vi "LEMP_realtime_theory_object_update.vi"() -> ()   [LabVIEW 2021]
uses:
  <vilib>/gmath/NI_Gmath.lvlib
  <vilib>/gmath/statdist.llb/Normal Moments.vi
panel:
  in  "Eigenvalue Method":u16(ring) items=["0-Local Eigen Modification Procedure", "1-LabVIEW generalized eigenvalues", "2-LabVIEW M^-1K eigenvalues", "3-LabVIEW Cholesky Factorization", "4-Cholesky Factorization CPU SGL", "5-Cholesky Factorization CPU FXP", "6-Cholesky Factorization FPGA SGL", "7-Cholesky Factorization FPGA SGL SCL"]
  in  "Width":dbl=0.0508 min=0.0 format="%#.6f"
  in  "Density":dbl=7900.0
  in  "Height":dbl=0.00635
  in  "Length of Beam":dbl=0.3525
  in  "Young's Modulus":dbl=209500000000.0
  in  "Torsion Spring":dbl format="%#.6f"
  in  "Initial Pin node":i32
  in  "Std. Dev.":dbl=0.5 min=0.0
  in  "FFT data length (data points)":i32=5000
  in  "Min. FFT Power Value (RMS)":dbl=0.02
  in  "accelerometer_mass":dbl=0.055
  in  "Std. Dev = Number of Particles / 3":bool
  in  "Number Of Particles":i32=5 min=3 step=1
  in  "FEA Nodes":i32=40 min=10 max=500 step=1
  in  "File name":i32
  in  "Auto FFT length":bool
  in  "scaling_factor_Hz_per_pin_to_frequency_resolution":dbl=0.33 caption="Scale FFT Factor" format="%#_13g"
  in  "Save Acceleration Data":bool
  in  "Max Roller Velocity":dbl=3.32
  in  "Bound to 1st Frequency":bool=TRUE
  in  "Mode Count":i32=3 min=1 max=10 step=1
  in  "Sub Sample":bool=TRUE
  in  "Bound Search":bool=TRUE
  in  "Frequency Method":T1(ring)=enum."FFT"
  in  "Truncate data length":i32=900000
  in  "Threshold":dbl=0.001 min=0.0 step=0.001
  in  "State Variance":dbl=0.004 min=0.0 step=0.001
  in  "Measurement Variance":dbl=0.02 min=0.0 step=0.001
  in  "Kalman filter":bool=TRUE
  in  "Loop":bool
  in  "MASTER":bool
  in  "Tab Control":enum32{"Real-Time Plotting", "Check"}(tab)
  in  "Pull Plot":bool
  in  "Plot Update Frequency":i32=1 min=1 max=120 step=1
  out "Cycle time (ms)":dbl=1645000.0
  out "1st Nat. Freq. (Hz) 2":dbl=51.5242069586 format="%#_5g"
  out "Acceleration Data":dbl[](graph)=[0.004838346699578007, 0.005707314680912377, 0.0002457456696160461, 0.00244141, 0.0035099822267943433, 0.0030151472637129956, 0.0013236796439387059, 0.0012207, 0.0004804562859344005, 0.0026911643741527698, -0.002564447036510659, -0.00244141, -0.003057944930129751, 0.0006807291071923737, -0.003240831363996899, -0.005531444031541692, -0.004714637474773665, 0.0010040428595001255, -0.000895050594271223, -0.005629411525551865, -0.008489750172548691, -0.009763279567137566, -0.0034487919855606085, -0.005997192514402743, -0.0062084927089418145, -0.009444646677602543, -0.005999196861104334, -0.007645857236281309, -0.0032866403259410966, -0.004668159383758392, -0.0032933255300085203, -0.005358923678449098, -0.00366211, -0.008061453273063023, -0.00484035189258754, -0.0045066733606962915, -0.0029596483182679945, -0.00646427838665329, -0.0028215566310879204, -0.0037774566118754767, -0.0002490891480864305, -0.0023180316433592464, -0.0006332527526784805, 0.0009438634648677151, 0.004850712645841344, -0.00025276350318602023, -0.0004557141195456918, -0.0006158703122225819, 0.0033728991099136883, 0.003753383579822631, 0.0055608666063529195, 0.0032692542591880543, 0.0016673890934073982, 0.006823699383774974, 0.0063806895946540085, 0.005189072881406364, 0.00610352, 0.005387679632948813, 0.005685583133382022, 0.006202820986014994, 0.006322851470832936, 0.0069310238098390445, 0.0065960097863841894, 0.004973752689676183, 0.008818081298295706, 0.007361332489712727, 0.007013946211991566, 0.007315861331160505, 0.0040763683073329155, 0.00474172038075455, 0.005847073938624507, 0.00707546550534147, 0.0039646969322940165, 0.004183356589966348, 0.0030492540591744847, 0.007616771509314835, 0.002959310243788487, 0.0022598558832947666, -0.0018462703396891047, -0.00033969769378417976, -0.0009769652177948614, -0.0024213458066581557, -0.0014106097343258841, -0.0034384320213449475, -0.003255874250872593, -0.002801167107613562, -0.005980145710809102, 0.000221340731292324, -0.004286669737069774, -0.001835568693656458, -0.008443278378544958, -0.00610352, -0.005691265776355962, -0.0034498018762239135, -0.008345314442677283, -0.00732422, -0.006807319917820242, -0.004058646874805149, -0.005983154182417148, -0.006446221826925894, -0.005471935187650813, -0.0020873291536892863, -0.006801634595950505, -0.008287138652413017, -0.00812162036147796, -0.0027132346534812545, -0.00213280168172932, -0.005811630805149362, -0.005547161177802966, -0.003514997126796511, -0.00018857387847851913, 0.0005807652314572483, 0.0, -0.002424358175864042, -0.0006713710325948414, 0.0007422551547140561, 0.001450402160948192, -0.00222876488360425, 0.002104050934057791, 0.00488281, 0.005521755058865002, 0.002690832678747488, 0.003996122407556653, 0.00580026125173535, 0.007844462402134508, 0.0021134087592309062, 0.0038884627526311107, 0.003656095075302359, 0.006979173442865501, 0.004359224886379336, 0.00610352, 0.006638127584099871, 0.009700756729686148, 0.006027615631327147, 0.0067083532785389335, 0.008215917923834175, 0.012035814637131893, 0.006443550649118248, 0.0038553632155707714, -0.0004941685208743052, 0.004581897304940234, 0.006142635343743659, 0.006208162207516742, 0.0031997099917495603, 0.00366211, 0.005981145420380271, 0.006130594642598011, 0.0013564458942844544, -0.0015269686304451436, 0.0006529809942469249, -0.00038149292787483403, 0.0008111245549630717, -0.0032257836072580727, 0.00022000106538775776, -0.0005272648315634695, 0.0011364443878150395, -0.0015697656312908224, -0.0012183645631356848, -0.00244141, -0.00366211, -0.00488281, -0.006871844272753541, -0.005599985746352319, -0.006023944820604123, -0.00737637483167438, -0.006316494754865866, -0.004697581898098994, -0.0018877239606148004, -0.004747405861413818, -0.00578287514930457, -0.006930024100267877, -0.005257279898645738, -0.00610352, -0.0060714159572628715, -0.007401788446975464, -0.00732422, -0.00610352, -0.004198067847207703, -0.002393932566436293, -0.0011795777649753398, -0.0018151735032415346, -0.0027299512489689045, -0.005892880805323408, -0.0017436240371379213, -0.0014487299534369866, 0.0017844128593840565, -0.0033264251711499337, -0.0008181465078102745, 0.00105520063282516, 0.006238927471955043, 0.00366211, 0.004266947017311713, 0.0034491284196068814, 0.00488281, 0.005911937740335157, 0.0023508003889117874, 0.0035718327963796767, 0.00488281, 0.006342575918813561, 0.006574943544279412, 0.005220837337713913, 0.0025577628292172, 0.008568656168129508, 0.008559965603939512, 0.008913035776453056, 0.00617239543133123, 0.005235883064907329, 0.00610352, 0.00488281, 0.005059345809346336, 0.005696616666619297, 0.006564245771016188, 0.0047062749137077005, 0.0042305006464292685, 0.006241267088496158, 0.005662178668874721, 0.005612696954273782, 0.0011755663981898382, 0.0022498235250871996, 0.00244141, 0.002234783141670752, -0.001692136877541692, -0.000652310517670898, -0.00033367806078744177, 0.002381227337734144, -0.0006135262941831664, -0.000622219309756346, -0.0028225630073968107, -7.756876469663552e-05, -0.003810557031028076, -0.004751416187353056, -0.004430773188134092, -0.005068038860597254, -0.005294059876738449, -0.005373635056169853, -0.00838810855109365, -0.002880742834804564, -0.0035460892961362003, -0.00305894561491835, -0.00488281, -0.005903244653513084, -0.005737738901643957, -0.0060322972801503515, -0.008480391076419833, -0.006561907318468658, -0.005380322662318899, -0.00366211, -0.0036728090961173957, -0.00395900739521185, -0.003067975817578463, -0.0033866082744263924, -0.0013069618159475523, -0.00244141, -0.002721588153838221, -0.00366211, -0.0012207, -0.002389245097183306, 0.00023872756780409714, 0.0020599131033494883, 0.0029081555984446683, 0.0014082723746651543, 0.0023641723555592924, -0.0007646500931260275, 0.004064327469096378, 0.00244141, 0.0033675474061745933, -0.001959949194888764, 0.004365909917820241, 0.0061700502765814035, 0.006349262202179489, 0.0036811678170329547, 0.007011940131482877, 0.006652177855351259, 0.006510752125436297, 0.0038045421062238532, 0.004760442087117992, 0.0058059457792666285, 0.004096762560982649, 0.00478150293344079, 0.0045019924869676604, 0.006842091980290595, 0.00610352, 0.00610352, 0.00366211, 0.005311111700909934, 0.004773144264601295, 0.00446487655710155, 0.0019138064995993128, 0.001969639797291477, 0.00011167227335184959, 0.002178611298253164, 0.0005814290057599253, 0.0033414714626078547, 0.0036560917420400793, 0.0018081546535116046, -0.0005356282963848078, -0.004769472078770399, -0.0023895858285402235, -0.0014818278498509277, -0.0022839270337424136, -0.00387508888250213, -0.00568090397158421, -0.00212143710766641, -0.00244141, 0.0004249534210508095, -0.004244875086274346, -0.004140225858656499, -0.005679564842518866, -0.003978068545613665, -0.0056768917939908695, -0.005728378583931971, -0.007064429539822786, -0.00488281, -0.006370663056698586, -0.0037112589728359154, -0.0033902886797810253, -0.00243906955354927, -0.00334113711587417, -0.0037206206820185727, -0.0033996477978572156, -0.00033702244852667866, -0.003383596083253921, -0.0033297679649829937, -0.00645859112548223, -0.0007700023774213725, 0.00036343492196830914, 0.0018425933279252694, -0.0016673947274447281, 0.0008930401807386253, 0.0029820468446669786, 0.002784780679218322, 0.0009177810134593685, -0.0021384882744482185, 0.0016650480497178732, 0.0023180290440713803, 0.003473538044353423, 0.001085960482131017, 0.0036216540427372636, 0.0042860035989600795, 0.006090146075020453, 0.00488281, 0.005459562875937074, 0.004624694305643805, 0.004822293237472738, 0.0023581507641239293, 0.0022665409312405795, 0.004070683407300953, 0.006752485176768145, 0.005748771640649356, 0.005634427660903092, 0.0044143914296922914, 0.00681968937004343, 0.0034150277485304127, 0.006883881922786926, 0.001413953215570771, 0.0032180956915600894, 0.0035226874034559553, 0.003437091673613087, 0.0001711858887514268, 0.003779463451115941, 0.0025049310133383467, 0.0051710218625556, 6.620083809203564e-05, 0.0006593345000990376, 0.0027861208819265834, 0.003613961988447113, -0.0010261096576971748, -0.004639743626408766, -0.00454780030398452, -0.0001999393590713065, -0.0003560802656662142, -0.002350129753546229, -0.0016854457956681078, -0.0032237802081354658, -0.002613932925239394, -0.00244141, -0.004060985677870505, -0.0005536797370022907, -0.004203749887713588, -0.005013545116369545, -0.00589588774036613, -0.0048443601232814795, -0.0030017751602588187, -0.0024875449465853045, -0.004579557493860795, -0.004867430049291275, -0.0018887275513499544, -0.0003988749850162539, -0.00366211, -0.004744390443728062, -0.0027149019993107284, -0.0018646602738848928, -0.0018074801561548896, -0.003292990175260752, -0.00020862961105360973, -0.0004603954807054018, -0.00028352720896955525, -0.0026008905040078886, -0.0009910078389807537, 0.002034841016163012, 0.002089675773720017, -0.003729311807663045, -0.0010986679348103173, -0.0001624896330411393, 0.004746396244896765, 0.00366211, 0.0018094895755103907, 0.0020923468857567207, 0.006044340462914497, 0.005221171687186573, 0.003378250369761096, 0.0029315623418507426, 0.00244141, 0.003314051815957536, 0.003044238844048012, 0.002058915746380744, 0.0029509554970910306, 0.003990772859533483, 0.003500952336341925, 0.0046079769679292885, 0.00678057069293091, 0.004440807685552677, 0.003676149268750784, -0.0005520051219315122, 0.003942625001398758, 0.0037754535496823975, 0.004537096894016044, 5.951396598845692e-05, 0.0015095779622130543, 0.0042923536784602685, 0.0046307177212724605, 4.8146129841106396e-05, 0.0006854136537807339, 0.0004573909422663496, 0.002200678364834297, 0.00228560377432933, -0.0025035919995941964, -0.00244141, -0.0016938075951212128, -0.00039519894277873424, -0.0009007338455109153, -0.0004517024650966952, -0.001087629991786761, -0.001406263968766161, -0.00214952115307032, -0.003264237362366076, -0.0034243888086113745, -0.001938878789398931, -0.00488281, -0.004006152810171153, -0.0036875203533232237, -0.0030278542071204657, -0.003053264560408162, -0.00366211, -0.0024129902930830516, -0.0005145624979940814, -0.0004443513831933158, -0.002677793155316665, -0.006830722843023242, -0.003644058559275936, -0.00244141, -0.0009127696302308469, -0.0023053297562428856, -0.0009094268967618322, -0.002320038463426881, -0.0002574480553589133, 0.0005697284251085758, 0.0022377869925913957, 0.00118058161320973, -7.48936729638779e-05, 0.0, -0.000754291670740479, 0.0, 0.0011785723089977865, 0.0012207, 0.0018252038838731748, 0.0004945035331790663, 0.004817278036147725, 0.00488281, 0.004570865455924278, 0.0043582218433327255, 0.002528005809353382, 0.00244141, 0.0021715880991365257, 0.00366211, 0.003802535636816153, 0.003505631958394223, 0.0032191005505475385, 0.0037864869926045324, 0.004050622519831631, 0.00488281, 0.005767498323731505, 0.002582504330283522, 0.002937580583412336, 0.002703204223548053, 0.003756063196485227, 0.0024079751876221853, -1.3037050029254208e-05, 0.0030007719528381436, 0.002722929967135202, 0.0035878847165482517, 4.8813368983473965e-05, 0.0, -0.0005376277156337268, 0.0032983399862966363, -0.0008031041934160126, -0.00244141, -0.0029666673267519294, -0.0004343176197846724, -0.00016951760067881062, -0.0004386629416658717, -0.0011006695152175844, -0.00039720557108254787, -0.0010759293810422067, -0.0020565737332359575, -0.004618006828262141, -0.0015145949330229013, -0.00366211, -0.0019860251438268725, -0.007237623988069004, -0.0018332257628127292, -0.0030953873706623964, 0.0007783647028999064, -0.004675514672692802, -0.0020813155957404806, -0.0033936306763945427, 0.00010398001093507863, -0.002250831569467771, -0.003227121481766, -0.003907188173045497, -0.0013902151931192378, -0.0002982385264328467, -0.0023614996303370005, -0.0032277935661562452, -0.0008736471213269573, 0.0024444157957709723, 0.0006880841660173035, -0.0007609763297872807, -0.0010351370446903465, 0.00045036297452209686, 0.0018659945220246212, 0.0006533162338866629, 0.0012046513557883794, 0.00244141, 0.001925508112879999, 0.00109131004111009, 0.0023956041194389058, 0.0051375862558038, 0.004098433705771313, 0.003443112875900749, -0.0005232510380810936, 0.003978067403567412, 0.004145909753484409, 0.005112513514073204, 0.0007673283154368679, 0.0031900123829050947, 0.0033705566749311286, 0.006656193360799982, 0.004283996661187547, 0.0010518591974529546, 0.003945973475725152, 0.005930996603656799, 0.00244141, 0.002959976565338493, -0.0002537665462326313, 0.0048717765270201874, 0.0009448665078077446, 0.0006800664887018826, 0.00012170441791931812, 0.004682201536579453, 0.0032933255300085203, 0.00046240282370421746, -0.0010060493837228655, 0.0010127363188584104, 0.0023942636455720587, -0.0016560273295690045, -0.004561168422371273, -0.00244141, 5.918156951199762e-05, -5.617374142111316e-05, -0.0012207, -0.002018125275235756, -0.0006904260476557334, -0.00037179359080780414, -0.00366211, -0.0027068813229235815, -0.003025513779807038, -0.004246882473309934, -0.004881472612923153, -0.004244207699227294, -0.0019138060476683349, -0.0012207, -0.00244141, -0.002068275965489608, -0.0013835325362636164, -0.0014310058313062118, -0.0013290292358210136, -0.004089070805240841, -0.003457485894288531, -0.0015336498438961385, -0.0031756341441363553, -0.002737973755133877, -0.0011344416350906783, 0.0012207, 0.0015774544481117867, -0.0006058375594248898, 0.0, -0.002197336069530328, 0.0029940807640734556, 0.0006322497124063724, -0.0006272370802049666, -0.0011956239522902994, 0.001794112032325712, 0.0030198298849436014, 0.003583870731337581, 0.00366211, 0.0028188874856001868, 0.0031375199424836433, 0.002647367600668428, 0.00454478450842671, 0.0060302945275325735, 0.0037497111365990808, 0.0021371532073547785, -0.00022166917012664267, 0.003928252068061328, 0.004912904623381627, 0.0055137307148118595, 0.0018817053383000672, 0.0029803769679529733, 0.002178609400036476, 0.00592564679816992, 0.004060314738443125, 0.001115380484902026, 0.0027506807477363266, 3.744691327983805e-05, 0.0017854189810747952, 0.0006466266228429885, 0.004627369079690917, 0.00244141, -7.522489182292804e-05, -0.0010404913613056043, 0.0006048349301412335, 0.0012207, 0.0003493923583009048, -0.0018656587099389783, -0.003366546258534641, -0.0012207, -0.0014684549547972687, -0.0024584550644151746, -0.001408603645564741, -0.0017673651027334805, -0.0006773865242249099, -0.0031589181347539616, -0.002521653220987049, -0.0037687643330156857, -0.0024149914982151315, -0.004272961520171581, -0.00370323476309916, -0.003329769326182824, -0.003173624724780854, -0.00244141, -0.002508948044360964, -0.003338124831647582, -0.0008937146480376625, -0.0010234354149402788, 0.0017132007807744492, -0.0042442104903145095, -0.0027379717857748762, -0.004165635036994708, -0.0005255945329761644, -0.0014537456422641334, -0.000412252892359776, -0.0019037789508908314, 0.002287941087320893, 0.0015176044042504696, 0.001023773955152224, -0.003340133196426414, 0.0019649612408072776, 0.0012561458284850494, 0.003097732829367463, -0.0011304262283161328, 0.0006733771213559845, 0.003392291432505386, 0.004389314190599248, 0.003733994552183081, 0.002782774434371096, 0.0032669105177496496, 0.004689891922762395, 0.0037878243796103253, 0.0013330441494733658, 0.003814575869632497, 0.00366211, 0.005564885907950802, 0.0032134148178314587, 0.004891844053730893, 0.003917885965481551, 0.004416061930999319, 0.004214116491383797, 0.005403395028755975, 0.004851381405115182, 0.0033749061380368888, 0.0024504323993540895, 0.002737641224305503, 0.00244141, 0.00244141, 0.0019790038428203404, 0.0007272061763921028, 0.002288947255574217, 0.0028723797316345893, 0.0013323735058553528, 0.0003771446836842806, -0.0020512262722411573, 0.001293255894346459, 0.00017453157753961153, -0.0025761517419882435, -0.003411681268249327, -0.0012919199753960728, -0.002885084869879488, 0.001955937187182966, -0.003931925883298503, -0.0032137464448334036, -0.0020956926239530486, -0.00244141, -0.004591259630214771, -0.004272292826633157, -0.004590925283481087, -0.00366211, -0.004192049605575055, -0.00366211, -0.003930588493624789, -0.0037426875677917873, -0.004061320024639717, -0.0022264191564440455, -0.00366211, -0.00244141, -0.004115149852102488, -0.0032130823089504172, -0.0034013184633962, -0.0015971759874068812, -0.002855327129594027, -0.00244141, -0.00442341630511587, 0.00147313783352711, 0.0005606995069925032, 0.0009311573212411267, -0.003502960572566538, -0.0002958968775718182, 0.0005894532592492364, 0.0012912524541747437, 6.218875102699918e-05, 0.0013989096851068595, 0.0022093678772576544, 0.003895818381269552, 0.0026112581511567546, 0.004479253467573693, 0.00488281, 0.005563882864904191, 0.0025801639030411487, 0.00366211, 0.0029994320185850213, 0.006820024061888043, 0.004690226269531608, 0.004288005499898549, 0.003613967269263169, 0.0037343288989167655, 0.006831390865512639, 0.006577952673206082, 0.0039991315283374506, 0.003717277365112223, 0.0042823232292121295, 0.0024755084388113353, 0.0021582159792129683, 0.00244141, 0.004174663574357642, 0.0025661168501571706, 0.0021381512516642958, 0.00026781248150797377, 0.003251194497456046, 0.002906147940179439, 0.002265876516017607, -0.0007913975952352189, -0.0018469352533701136, -0.0012207, 0.002076302347340614, -0.0020475479101623394, -0.00244141, -0.0016072080142339252, -0.002237792270597422, -0.0012207, 0.0001638305806441879, -0.001330702807484188, -0.0024835378060391895, -0.005801265543683791, -0.004908559805578524, -0.005929989465948213, -0.0026403466447372974, -0.004165970558713408, -0.0028516479211006867, -0.005428472059686869, -0.003755727091187084, -0.0032659090961410803, -0.002931227995081531, -0.00366211, -0.0027363038372997103, -0.0054598986798768435, -0.00479555192551951, -0.005751451906307066, -0.0028439634921541986, -0.00244141, -0.0007643198110321677, -0.0023143577129785143, -0.0017309152369181413, -0.001147482760928823, -0.0003283285127287439, -0.00244141, -0.0030442346671812406, -3.443771570114181e-05, 0.00039720169550309524, -0.001088298323709348, 0.0008579337715701141, 0.00229930704741205, 0.004220801618759902, 0.0003918551985566607, 0.00244141, 0.003412352974518827, 0.004215452511605226, 0.002593203426436445, 0.0018817073870183061, 0.0020839868556818686, 0.003549100797051287, 0.00569227180773156, 0.004710625716208068, 0.003952660424520048, 0.00732422, 0.008026013837276025, 0.0071951568885285175, 0.00366211, 0.003672809139941006, 0.005163668707212147, 0.004294025365672687, 0.002711562177479383, 0.0024898902794040735, 0.005002178783848758, 0.0055685608107389345, 0.003878432350052139, 0.002850651265309703, 0.004040924872641506, 0.0034394311201956062, 0.0022789161462684797, -0.0018168477047625213, 0.0010170889373351424, 0.0012207, -0.00021732628049132445, -0.0003808192330379766, 0.0012207, -0.0009475425827972237, 0.001056200947709941, -0.0009569004108514229, -0.0006382679539679666, -0.001540338115580733, -4.0121693053591295e-06, -0.00212377798136181, -0.003129490832648443, -0.004351198660685468, -0.0024942367871906633, -0.0037684292248823053, -0.0031315017009220488, -0.003026180736799389, -0.0016473282059380765, -0.0036069393016254976, -0.003394966943301414, -0.003503963985197222, -0.004304057082888904, -0.0043578895206665, -0.003758398794949104, -0.008023338208739572, -0.0034477937304920776, -0.002974358726391379, -0.002328059474111163, -0.0012711867734980814, -0.003393963903029306, -0.00244141, -4.0458540045694305e-05, -0.002438066505060235, -0.0012207, -0.00244141, -0.0014821613037496136, -0.0011635267049872199, 0.0008448942481392907, 0.0012207, 0.0010130706655565678, 0.001553710276553398, 0.00244141, 0.0003931895235298145, 0.0032007102191292307, 0.0034972770501327318, 0.0004593903614086873, 0.000488815242401863, 0.00366211, 0.0047915397534396475, 0.0051278905724236705, 0.00488281, 0.0015436797205917907, 0.003792837348705732, 0.005512390095850358, 0.006990205045196016, 0.002472169964484943, 0.0026831400300996273, 0.0035929002218640315, 0.00366211, 0.00256444960559874, 0.00366211, 0.0043608947165307554, 0.005900235508081506, 0.0029028094658530464, 0.0035808601835860114, 0.0031940245439579995, 0.003064296778901612, 0.0015590603013004357, 0.0007328880854626855, 0.0004363259080498222, 0.003088369402918144, 0.0008920389673632576, 0.0008084493262815332, -0.00027884928785664636, 0.0035785229690199357, 0.0028315903943899826, 0.000506200742222478, -0.00213481151467014, -0.002417336935079447, 0.00012671929316412402, -0.0030128086031098993, -0.0029469422925239392, -0.0035962436893785133, -0.00244141, -0.00244141, -0.0016456614652801062, -0.0005984826511725647, -0.00331806718979332, -0.0012685129829208535, -0.005523091657081342, -0.005582940682043727, -0.0051579673788754495, -0.0028513191207926395, 0.0004904851929616282, -0.007719414138544437, -0.004625367471893895, -0.0027463284060027134, 0.003362534387848679, -0.0028185508354235302, -0.003104419786308231, -0.005208468786613705, -0.0024741759819616647, -0.002225749087939859, -0.001701160931166003, -0.0017175413119385934, -0.0023009837879989664, -0.0003888452752560057, -0.00019425546427892407, 0.0012207, 0.00244141, 0.0008853538317702245, 0.0016800962037858001, 0.0002815211202794666, 0.0025948722459413864, 0.0019860237879628846, 0.00040957477405895474, -0.0018328967707408608, 0.002735298898988549, 0.0032318012188197473, 0.006434517523935618, 0.0024745103286598225, 0.0043117457436237855, 0.0042786454149639636, 0.004614000328742904, 0.0013036183347026652, 0.0006787266913620145, 0.0023461157846983586, 0.004638736869382263, 0.00244141, 0.004055301783078122, 0.0039680414489427435, 0.00488281, 0.003918889359081515, 0.0032150883894946332, 0.004117155932646704, 0.0032528684552082026, 0.0007288774170804407, -0.0002189971240637242, -3.410679535490813e-05, 0.0034143583784650103, 0.0031900104491883047, 0.001552710870937469, 0.0005162342344014804, 0.00366211, 0.0034334144452570145, 0.0012133493563682477, -0.0015142588551145145, -0.0035868817748082116, -0.0012207, -0.0012207, -0.00244141, -0.003583204165983217, 0.00042562341827057527, -0.0015135918898697093, -0.0010348032045960978, 0.0, -0.00013340805259954213, -0.0018028013914374887, -0.003794176967976658, -0.008273093032048817, -0.003241500060203244, -0.0040890708052763675, -0.002676122062461956, -0.005141934796016884, -0.00244141, -0.0017553276499418671, 0.0011230705478503175, -0.0009264748562031861, -0.0018385778225831278, -0.00244141, -0.00244141, -0.005235884469895242, -0.004328797428107514, -0.0029559677267340734, 0.00185864156111291, -0.0004169304026263416, -0.0020007350753684983, -0.0013521052997685994, 0.0032508623692215624, 0.0027506770145480793, -0.0010110682415448084, -0.004244206652938606, -0.00019091199669338818, 0.002133472465070617, 0.0021351419418586533, -0.0032926556259139255, -0.00048647252260136534, 0.00262930826080972, 0.0035280341769678737, 0.004822627419867885, 0.001194289052380954, 0.0005897926184504202, 0.0018716807970934018, 0.0036283409778017544, 0.00244141, 0.0037834778718592622, 0.0054104172857005264, 0.0026166076992509796, 0.0020331659408732742, 0.003204053070374197, 0.007836103429162137, 0.0045999526458945315, 0.0016807649027666476, 0.001768029257789296, 0.0025647839523679516, 0.0018064771131082787, 0.0029553009613634343, 0.002385232925210026, 0.00373165412490518, 0.005356252963528332, 0.0040593132456922445, 0.0005520064913482695, -0.0011421283840561014, 0.0039830854396256145, 0.00244141, 0.0010388207696834348, -0.0035096475678174375, -0.0020846590906447183, -0.00013006088743244175, 8.726264597291389e-05, -0.0022575185318864906, 0.0, -0.0014584265159927642, -0.0003457159600676087, -0.0021498584360569273, -0.00197699855384008, -0.0019114668091058547, -0.0005951391728798161, -0.003063293327925269, -0.002809855877845579, -0.0025798232675128515, -0.0023762118488166906, -0.0010137414352029864, -0.002594536127019419, -0.0008906997534962515, -0.00243004211721901, -0.003055939334455275, -0.001815507748562067, -0.0018890668995241813, -0.0013480864612707604, -0.0020803125472514455, -0.0042030830484616625, -0.00332642221586629, 0.0008355317502382353, 0.0007817059133918927, 5.685913452943992e-06, -0.0007151663269968193, -0.0016907990770926883, 0.0010351437113214862, 0.00027483593253931505, 0.0009913381265525647, -0.0008127969597515766, 0.000698116023027859, -0.0013029561928294597, -0.001098997781407053, 0.002699191347586983, 0.0031535638647012887, 0.004475245971067329, 0.0012207, 0.0009348360777679619, 0.0017713739413379001, 0.0005436500492959563, 0.003474875434027136, 0.0002410670036083495, 0.00107325747740602, 0.0008719781209785706, 0.004480255683343084, 0.0028606808299042425, 0.0034070034264956565, 0.0026055742563643723, 0.0035076417995164428, 0.0011448071623079395, 0.0012207, 0.001551704190673339, 0.003841318153886544, 0.0017476348014198399, 0.001691132810153725, -0.0009946811312156931, 0.002613596431148821, 0.00244141, 0.0035975784442642588, 1.0699118100254853e-05, 0.0021254497288316922, -9.696095588855808e-05, -0.0013373913995223493, -0.0021856338947951657, -0.003033869419197385, -0.002377546688681735, -0.0006409444782205022, 0.0022314393782758486, 5.01554834611926e-05, -0.00026379958914857704, -0.0010608822514222177, 0.0021237792824462852, -0.0014865117584356034, -0.0031843250095070887, -0.00244141, -0.0012758706983745025, -0.0022264206846858616, -0.00244141, -0.0035056352916565023, -0.0010658996357463296, 0.0, 0.0018074859573052598, -0.002436394784980109, -0.0009609151958074481, -0.00063893664750639, 0.0006944382087086385, -0.0023304064228544955, -0.00366211, -0.0019134721501266527, -0.0002093010681829095, 0.0013300322843100485, 0.0015854788030853046, 0.0007465963023608783, 0.00228593748562067, 0.0003263237688046318, 0.000996025034315548, -0.00042027387017635044, 0.002136484927366147, -0.0011394601834794306, 0.0002989072227102458, -0.001463439739670796, 0.005721026138054258, 0.0016249296630341855, 0.0029472762969567257, -0.0008485743795963612, 0.0060553739193183465, 0.006025614546674468, 0.0039255757819220355, 0.00051757089561426, -0.001041155302650267, 0.00421111116942008, 0.0019178186935199255, 0.0022364537606116234, 0.0014480567242259853, 0.00244141, 0.004413052810182995, 0.003045910169893284, 0.004045270008201309, 0.00391052963847538, 0.005633421648700324, 0.0011234050944936955, -0.0005566855327732629, -0.0006576633361375442, 0.0033000124650730107, 0.0034013188193919765, -0.001735933840015351, 6.620092854928497e-05, 0.0015413435879921401, 0.00602060175020558, -0.0007964185783601364, -0.0004985157052589282, -0.004322448586659834, -0.00012838967957628416, -0.0003828270336944115, -0.0018947515637910781, -0.005100476450358238, 0.0, -0.0011314358395328695, -0.00046541068203041503, -0.0018542946945915681, 0.0007051358970636182, -0.0009699459161694804, -0.0032645717091352878, -0.0035691616022802855, -0.0018977540262997707, -0.0017650209750639855, -0.002651709969827324, -0.007089507937538044, -0.0005590300629655927, -0.0005493315174269907, 0.0021424990221541747, -0.0012059887427941722, -0.0017747198411337897, -0.0013872100247513193, 0.0011909490414181818, -0.0012892416461230747, -0.0032749364584834717, -0.0008967237770709136, -0.002048885302646083, 0.0002447428266567648, 0.00010231371954016457, 0.0013831962996722791, 0.004597946565279262, 0.0031335063379905846, -0.000956906357203028, -0.00040623130643789183, 8.860188989759771e-05, 0.0027419858477834447, 0.0004252935661603614, 0.0012207, -0.000977294993249285, 0.004400352982740776, 0.004248893489417169, 0.004283660616288976, 0.0024985834510988635, 0.004545119778124126, 0.003005787321276197, 0.0017041733935681147, 0.00021866337446225246, 0.0016583666940533093, 0.00011133583389868031, 0.0020575783538970003, 0.00038015329771906017, 0.0033321097534607246, 0.0038115667405992457, 0.004606639580923495, 0.00244141, 0.00244141, 0.0012086668173424376, 0.002104387091112254, -0.0019726539304331914, 0.0005530095316203776, 0.00034905801149616596, 0.0012207, 0.0, 0.0018205230484902026, -3.978484520883734e-05, 0.002371196989828103, -0.0008786632703375361, 0.0014219821583995123, -0.001958611309247299, -0.0012207, -0.000791736357197608, -0.0005958042097792006, -0.004695241470821093, -0.005579262141824912, -0.00025677567515930075, 0.0003159576828008168, 0.0017727143000611898, -0.001516938195033991, -0.0012969351847959046, -0.002042865404004237, -0.0003196361517707383, -0.0022026844618123673, -0.0031047539605575055, -0.004193386992580848, -0.00244141, -0.0021488541933745208, -3.3434813159413657e-06, 0.0, 0.0, -0.000709488137419606, 0.0005556843056674901, -0.0007465963024319323, 0.0030910444069326276, -0.0016409805916225298, -0.0027262675458165665, -0.0041499204136142, 0.001628945168482907, 0.0015333204957929663, 0.0015453570282177157, 0.0016088776417722025, 0.002252168186821414, 0.002646360399892348, 0.003306027477346818, 0.00022668771840881352, -0.000977629909618845, 9.729490554183135e-05, 0.0005399700082250812, 0.0011989674609604699, 0.000593802267898206, 0.0030569423746918557, 0.0017937726842225396, 0.003694207288423241, 0.0048691060367309505, 0.0038981597754769023, 0.005462571553039347, -0.0017539909611616967, -0.0016252628868944456, -0.0011284239934358006, 0.0058932114956667435, 0.0025811669433132567, 0.0012257164666962233, 0.00033100419077992113, 0.0026915013722859115, 0.004108461331171111, 0.0021685756366278328, 0.0016617101752981962, -0.002085329539795462, 0.001204322955299718, -0.0004774518022393334, -0.0016800979458453508, -0.0024240238263558544, 0.0006024953190780684, 0.0, -0.001312650734056755, 0.00225919042185416, 0.0008656237469067127, -0.0012608250534214102, -0.004197731629753667, -0.004611988389458775, -0.002044537102314667, -0.0014794884277770808, -0.00244141, -0.003373901917301814, 0.00012772287877659775, 0.0015627431306484952, 0.0008586014762672833, -0.004717982185889662, -0.002253835702538431, -0.00244141, 0.0008194827992613449, -0.004379283788020277, -0.004152601361312368, -0.0005573560394424945, -5.215820054334326e-05, -0.0024397357627657487, -0.0005964746096994378, 0.0005556865817207058, 0.002237457811530209, -0.0005018544782402459, -0.0016279387920674362, -0.0025420447028289784, 0.0009368388303857417, -0.00041325258834264817, -0.00024574886881062854, -0.0003697861162315772, 0.0012207, 0.0022608589263413774, 0.0027078807996818222, 0.0013370536236622388, 0.0004045612297786665, 0.0022782445166902965, 0.0020602515776483826, 0.0012832233552599194, 0.0005122213256792843, 0.0019378790797211806, 0.002768735472492163, 0.0036534169843912933, 0.0018405814215088478, 0.003625666203754642, 0.004335818709941216, 0.004837673188145935, 0.002805179268701994, 0.002297300958650907, 0.0012207, 0.00029690072858071063, 0.00327660819232953, 0.003410346893974611, 0.0040536286907712086, 0.0003055941851289653, 0.0011364484797380392, 0.002512619386480787, 0.004658797674575735, 0.004863758849598185, 0.0007101511119769277, 0.0002865382553567967, -5.8176335249360994e-05, 0.0012207, 0.0005165704793518532, 0.00032297896467004607, -0.0024240238974981665, -0.0009428604218211043, 9.02739933987839e-05, -0.0005383004792899263, 4.9483319640654345e-05, 0.00011634965481550647, -0.00190745385922797, -0.0028720486195600615, -0.0034554828594496813, -0.002863355603951355, -0.0017008258723697108, -0.0038235994823172595, -0.006695646814558778, -0.00217225476031951, -0.0012788798275143347, -0.0004306395015102121, -0.0030291898658326402, -0.002279914856220128, -0.00488281, -0.0026028999233633893, -0.006000202514359188, -0.003554449904099382, -0.0014855100192124435, -0.0012207, -0.0006372675239660363, -0.0011130451246233923, -0.002176605201314709, -0.0024952398274445354, -0.0040345722843056694, -0.004353204741166804, -0.003451137198027935] caption="Accelorometer data"
  in  "Real-Time plotting":bool
  out "Probability Density Function":cluster{i32[], dbl[]}(graph)={[9, 10, 11, 12, 13, 14, 15, 16, 17, 18, 19, 20, 21, 22, 23, 24, 25, 26], [0.09171563397251428, 0.12108231855717679, 0.143041857841436, 0.1512135165862316, 0.143041857841436, 0.12108231855717679, 0.09171563397251428, 0.062165735159412254, 0.03770542435775916, 0.020464524096401888, 0.009939041952144324, 0.004319489826678621, 0.0016798304322918924, 0.0005845793791312176, 0.00018203990329545533, 5.072648364839732e-05, 1.2648760741233286e-05, 2.8223200098705454e-06]}
  out "FFT":dbl[](graph)=[1.1522251336885276, 1.1178137375595425, 0.22252534672789437, 0.009332931918381289, 0.043862184342658705, 0.020464933055920162, 0.00777523899540152, 0.006561779609540276, 0.009100710608339503, 0.01457300652644379, 0.017722707537955747, 0.007669972094880839, 0.021547173708648927, 0.030187487612448695, 0.02011379991274781, 0.005972128055311526]
  out "Frequencies":dynamicdata(graph)=[{"t0"=timestamp(0 s since 1904-01-01), "dt"=1.0, "Y"=array[8870 elements]}, {"t0"=timestamp(0 s since 1904-01-01), "dt"=1.0, "Y"=array[8870 elements]}]
  in  "PDF":bool
  out "Absolute position":dynamicdata(graph)=[{"t0"=timestamp(0 s since 1904-01-01), "dt"=1.0, "Y"=array[8870 elements]}, {"t0"=timestamp(0 s since 1904-01-01), "dt"=1.0, "Y"=array[8870 elements]}]
  out "Frequency space":waveform(dbl)[](graph)=[{"t0"=timestamp(0 s since 1904-01-01), "dt"=0.005584330543933054, "Y"=array[8870 elements]}, {"t0"=timestamp(0 s since 1904-01-01), "dt"=0.005584330543933054, "Y"=array[8870 elements]}] caption="1st Nat. Freq. (Hz)"
  out "Position Pinned Boundary condition":waveform(dbl)[](graph)=[{"t0"=timestamp(0 s since 1904-01-01), "dt"=0.005584330543933054, "Y"=array[8870 elements]}, {"t0"=timestamp(0 s since 1904-01-01), "dt"=0.005584330543933054, "Y"=array[8870 elements]}] caption="Beam Boundary condtion"
  out "average cycle time (s)":dbl=0.005584330543933054 format="%0.6f"
  # "Note: All Inputs are based on base SI units."
  # "the martian andy weir in german"
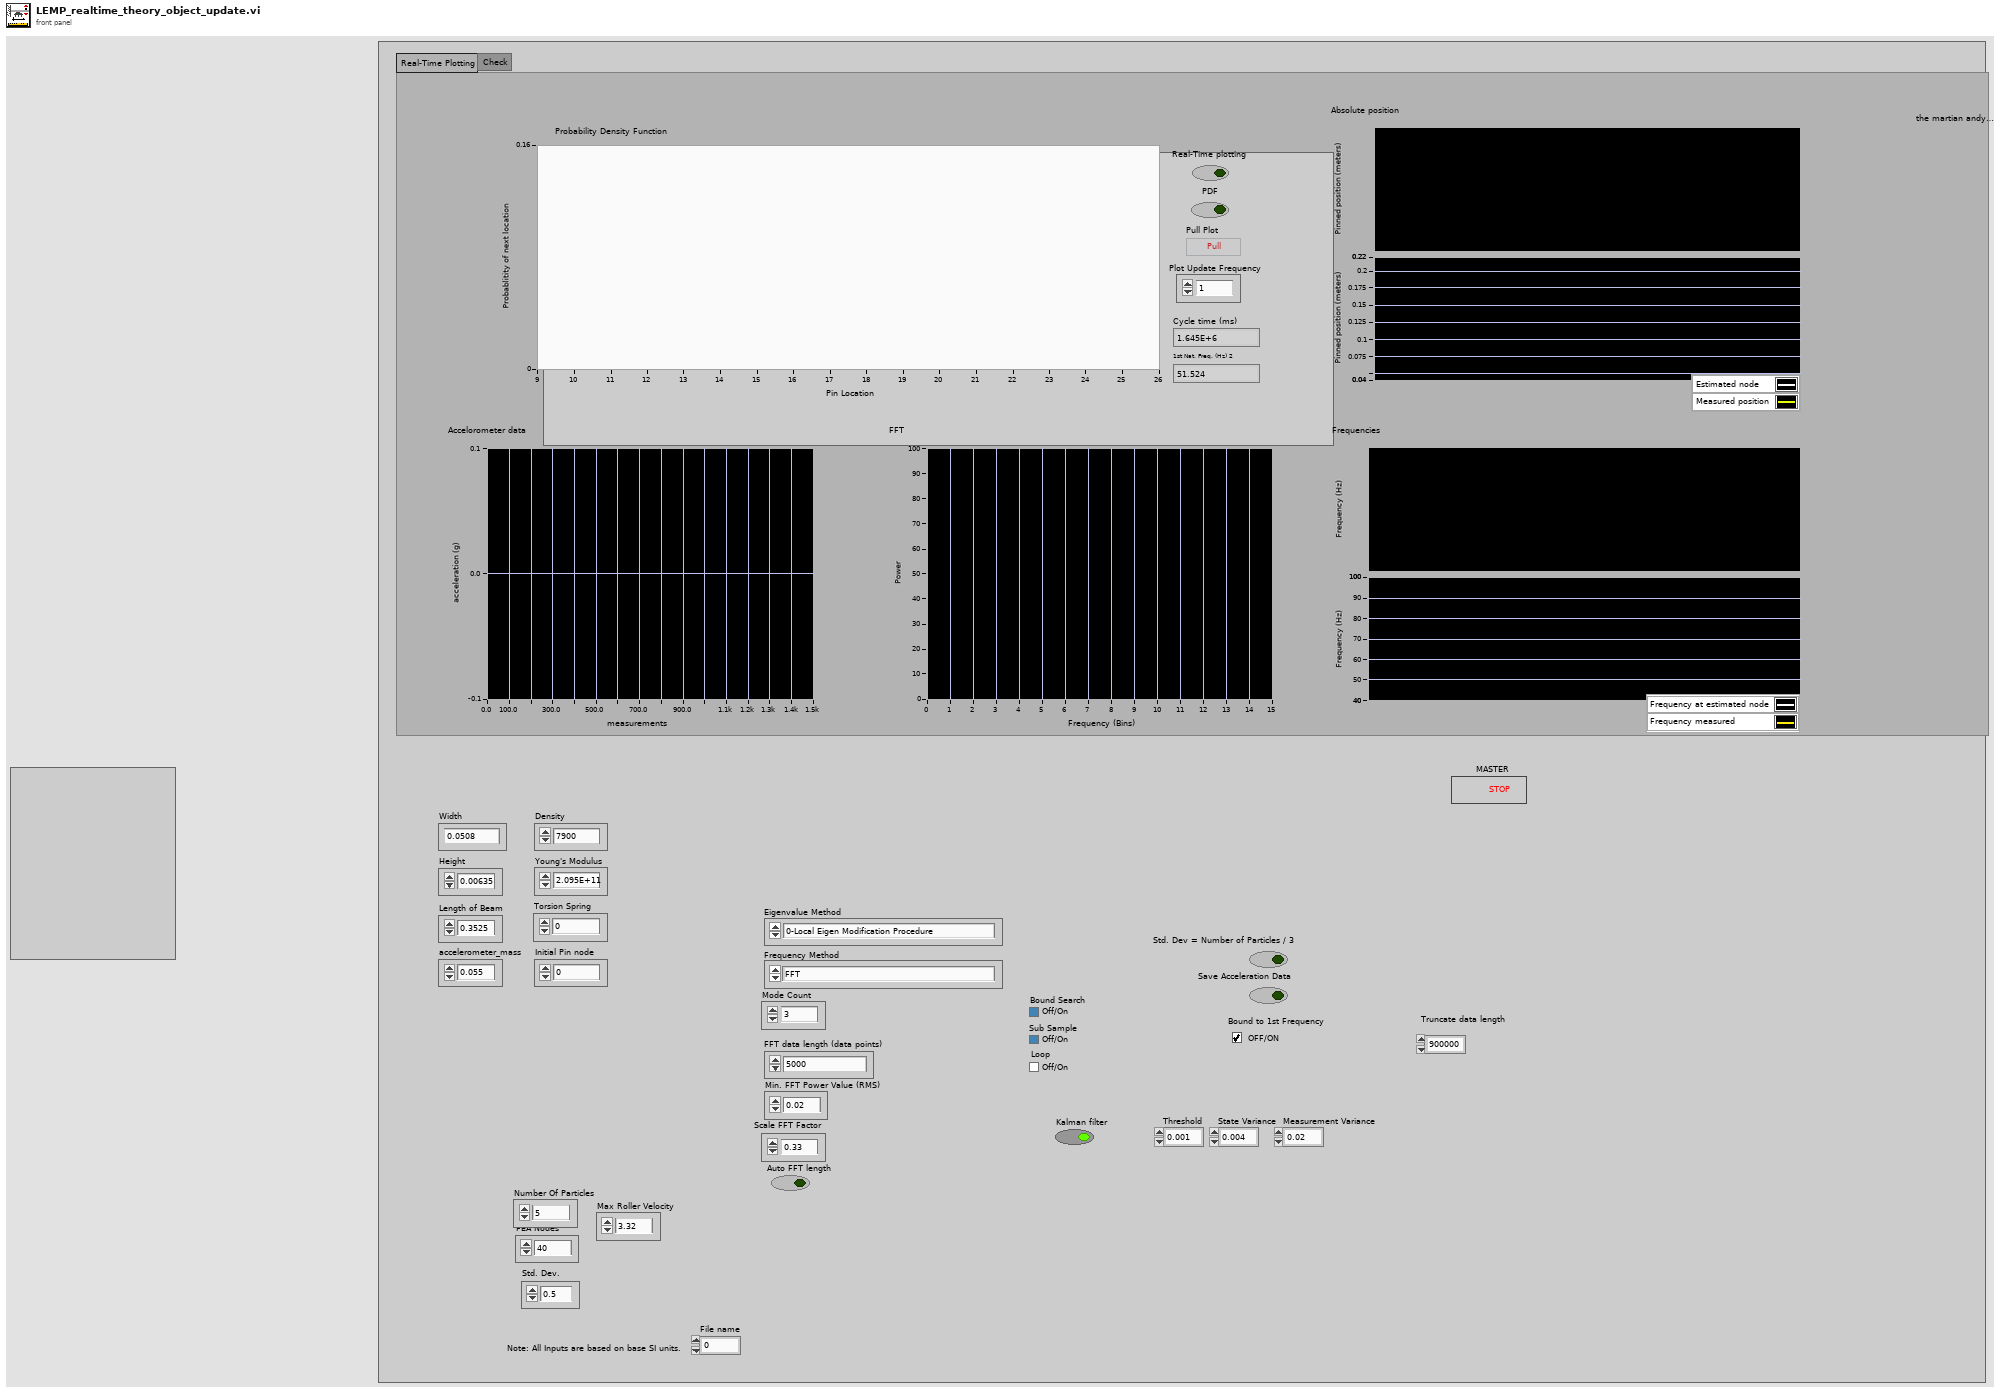
[diagram p1: front panel]
types:
  T1 = enum16{"Bandpass FFT", "Tone", "FFT", "Custom Filter"}
  T2 = cluster{"State":dbl[][], "F state prop matrix":dbl[][], "H measure matrix":dbl[][], "P process cov":dbl[][], "R measure cov":dbl[][], "Q state cov":dbl[][], "T Sample":dbl, "New Measurement":dbl, "Measurement Variance":dbl, "State Variance":dbl, "Threshold":dbl, "Initialized":bool}
  T3 = cluster{"Experimental Replay":cluster{"Accelorometer":dbl[], "Displacement":dbl[], "dt":dbl, "Final Time":dbl}, "Experimental Results":cluster{"time_average_cycle":dbl, "measured_frequency":dbl[], "date_time":string, "estimated_pin_node":i32[], "time_cycle_start":dbl[], "measured_pin_location":dbl[], "estimated_frequency":dbl[], "acceleration_data":dbl[], "accelerometer_sample_rate":dbl, "displacement_sample_rate":dbl, "time_compare_start":dbl[], "time_subsample_start":dbl[], "time_FEA_start":dbl[], "time_FEA_end":dbl[], "time_cycle_end":dbl[], "time_accelerometer_aquire_start":dbl[], "time_frequency_calculations_start":dbl[], "time_frequency_calculations_end":dbl[], "measured_pin_location_tt":dbl[], "time_ACC_data_collection_start":dbl, "time_acceleration_data":dbl[], "estimated_pin_location":dbl[], "scaling_factor_Hz_per_pin_to_frequency_resolution":dbl, "Std_Dev_equale_particles_divided_3":bool, "Auto_FFT_length":bool, "windowed_acc_data":dbl[][], "FFT":dbl[][]}, "FEA Parameters":cluster{"LEMP":cluster{"Eigenvalues":dbl[], "Square Transpose Eigenvectors":dbl[][], "1/deltaStiff":dbl}, "nodes of interest":i32[], "all nodes":i32[], "Eigenvalue Method":enum16{"0-Local Eigen Modification Procedure", "1-LabVIEW generalized eigenvalues", "2-LabVIEW M^-1K eigenvalues", "3-LabVIEW Cholesky Factorization", "4-Cholesky Factorization CPU SGL", "5-Cholesky Factorization CPU FXP", "6-Cholesky Factorization FPGA SGL", "7-Cholesky Factorization FPGA SGL SCL"}, "Mode Count":i32, "initial_pin_node":i32, "Sub Sample":bool}, "Modeling Parameters":cluster{"beam_length":dbl, "youngs_modulus":dbl, "torsion_spring":dbl, "beam_height":dbl, "beam_width":dbl, "beam_density":dbl, "number_of_FEA_nodes":i32, "FFT_data_length":i32, "standard_deviation":dbl, "number_of_particles":i32, "min_FFT_power_value":dbl, "initial_pin_node":i32, "accelerometer_mass":dbl, "Max Roller Velocity":dbl, "Max frequency delta per second":dbl, "Max frequency delta per node":dbl, "Min frequency":dbl, "Max frequency":dbl}}
  T4 = cluster{"time_average_cycle":dbl, "measured_frequency":dbl[], "date_time":string, "estimated_pin_node":i32[], "time_cycle_start":dbl[], "measured_pin_location":dbl[], "estimated_frequency":dbl[], "acceleration_data":dbl[], "accelerometer_sample_rate":dbl, "displacement_sample_rate":dbl, "time_compare_start":dbl[], "time_subsample_start":dbl[], "time_FEA_start":dbl[], "time_FEA_end":dbl[], "time_cycle_end":dbl[], "time_accelerometer_aquire_start":dbl[], "time_frequency_calculations_start":dbl[], "time_frequency_calculations_end":dbl[], "measured_pin_location_tt":dbl[], "time_ACC_data_collection_start":dbl, "time_acceleration_data":dbl[], "estimated_pin_location":dbl[], "scaling_factor_Hz_per_pin_to_frequency_resolution":dbl, "Std_Dev_equale_particles_divided_3":bool, "Auto_FFT_length":bool, "windowed_acc_data":dbl[][], "FFT":dbl[][]}
  T5 = cluster{"LEMP":cluster{"Eigenvalues":dbl[], "Square Transpose Eigenvectors":dbl[][], "1/deltaStiff":dbl}, "nodes of interest":i32[], "all nodes":i32[], "Eigenvalue Method":enum16{"0-Local Eigen Modification Procedure", "1-LabVIEW generalized eigenvalues", "2-LabVIEW M^-1K eigenvalues", "3-LabVIEW Cholesky Factorization", "4-Cholesky Factorization CPU SGL", "5-Cholesky Factorization CPU FXP", "6-Cholesky Factorization FPGA SGL", "7-Cholesky Factorization FPGA SGL SCL"}, "Mode Count":i32, "initial_pin_node":i32, "Sub Sample":bool}
  T6 = cluster{"beam_length":dbl, "youngs_modulus":dbl, "torsion_spring":dbl, "beam_height":dbl, "beam_width":dbl, "beam_density":dbl, "number_of_FEA_nodes":i32, "FFT_data_length":i32, "standard_deviation":dbl, "number_of_particles":i32, "min_FFT_power_value":dbl, "initial_pin_node":i32, "accelerometer_mass":dbl, "Max Roller Velocity":dbl, "Max frequency delta per second":dbl, "Max frequency delta per node":dbl, "Min frequency":dbl, "Max frequency":dbl}
  T7 = typedef "Control 1.ctl" = cluster{"Experimental Replay":cluster{"Accelorometer":dbl[], "Displacement":dbl[], "dt":dbl, "Final Time":dbl}, "Experimental Results":cluster{"time_average_cycle":dbl, "measured_frequency":dbl[], "date_time":string, "estimated_pin_node":i32[], "time_cycle_start":dbl[], "measured_pin_location":dbl[], "estimated_frequency":dbl[], "acceleration_data":dbl[], "accelerometer_sample_rate":dbl, "displacement_sample_rate":dbl, "time_compare_start":dbl[], "time_subsample_start":dbl[], "time_FEA_start":dbl[], "time_FEA_end":dbl[], "time_cycle_end":dbl[], "time_accelerometer_aquire_start":dbl[], "time_frequency_calculations_start":dbl[], "time_frequency_calculations_end":dbl[], "measured_pin_location_tt":dbl[], "time_ACC_data_collection_start":dbl, "time_acceleration_data":dbl[], "estimated_pin_location":dbl[], "scaling_factor_Hz_per_pin_to_frequency_resolution":dbl, "Std_Dev_equale_particles_divided_3":bool, "Auto_FFT_length":bool, "windowed_acc_data":dbl[][], "FFT":dbl[][]}, "FEA Parameters":cluster{"LEMP":cluster{"Eigenvalues":dbl[], "Square Transpose Eigenvectors":dbl[][], "1/deltaStiff":dbl}, "nodes of interest":i32[], "all nodes":i32[], "Eigenvalue Method":enum16{"0-Local Eigen Modification Procedure", "1-LabVIEW generalized eigenvalues", "2-LabVIEW M^-1K eigenvalues", "3-LabVIEW Cholesky Factorization", "4-Cholesky Factorization CPU SGL", "5-Cholesky Factorization CPU FXP", "6-Cholesky Factorization FPGA SGL", "7-Cholesky Factorization FPGA SGL SCL"}, "Mode Count":i32, "initial_pin_node":i32, "Sub Sample":bool}, "Modeling Parameters":cluster{"beam_length":dbl, "youngs_modulus":dbl, "torsion_spring":dbl, "beam_height":dbl, "beam_width":dbl, "beam_density":dbl, "number_of_FEA_nodes":i32, "FFT_data_length":i32, "standard_deviation":dbl, "number_of_particles":i32, "min_FFT_power_value":dbl, "initial_pin_node":i32, "accelerometer_mass":dbl, "Max Roller Velocity":dbl, "Max frequency delta per second":dbl, "Max frequency delta per node":dbl, "Min frequency":dbl, "Max frequency":dbl}}
  T8 = cluster{dbl, "FFT":dbl[], "Dynamic Data":dynamicdata, "Dynamic Data":dynamicdata, "acceleration_data":dbl[], dbl, "Dynamic Data":dynamicdata}
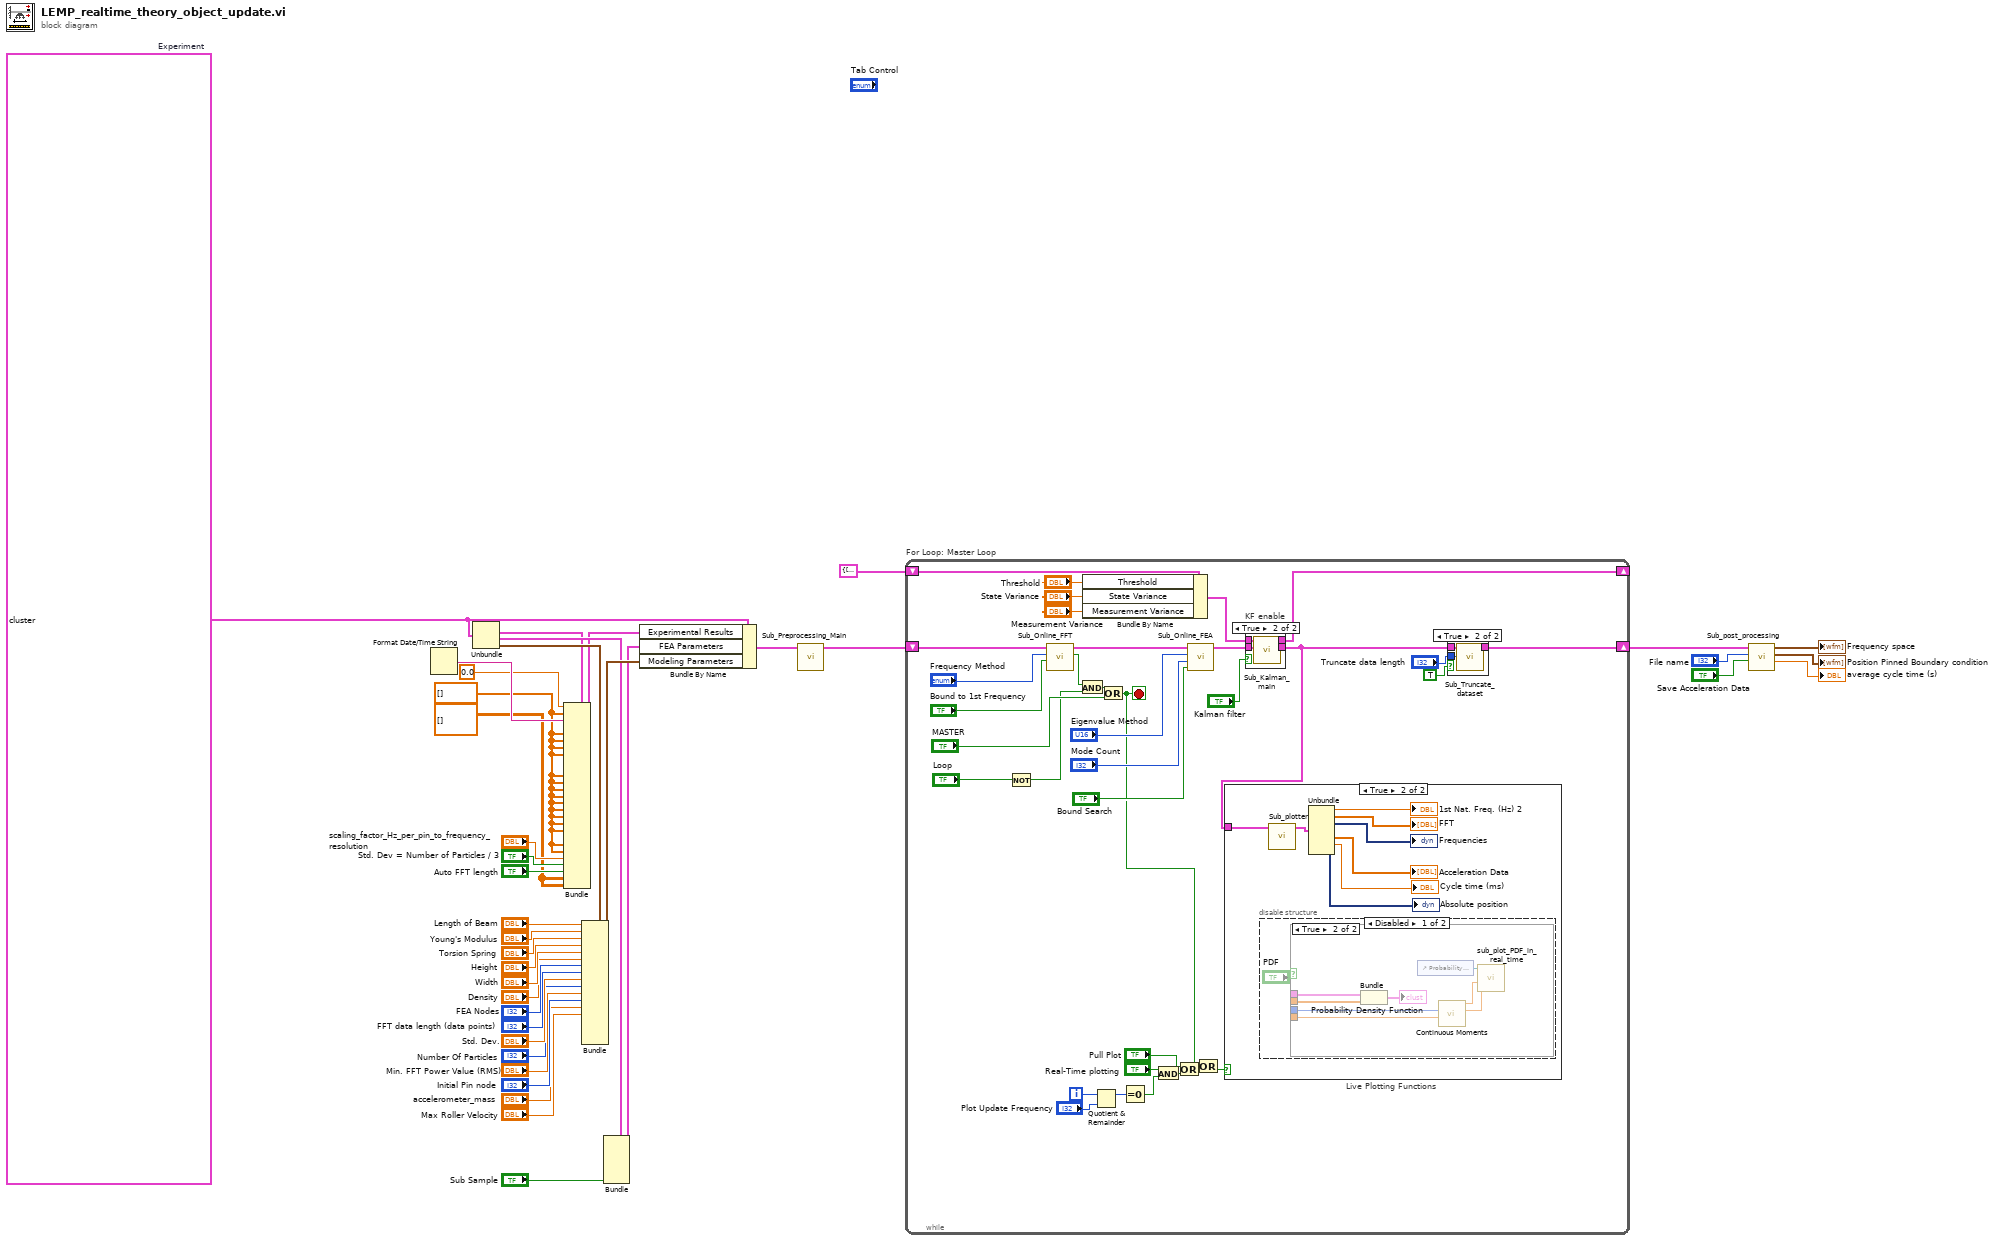
[diagram p0: block diagram]
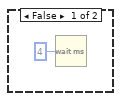
[diagram p5: hidden frame]
diagram:
  w3 = dbl[][] [] ("estimated_pin_location")
  w1 = dbl[] [] ("estimated_pin_location")
  w35 = T3 {"Experimental Replay"={"Accelorometer"=array[210000 elements], "Displacement"=array[210000 elements], "dt"=0.0002, "Final Time"=42.0}, "Experimental Results"={"time_average_cycle"=0.0, "measured_frequency"=[], "date_time"="5/2/2024 1:10:00 PM", "estimated_pin_node"=[], "time_cycle_start"=[], "measured_pin_location"=[], "estimated_frequency"=[], "acceleration_data"=[], "accelerometer_sample_rate"=5000.0, "displacement_sample_rate"=5000.0, "time_compare_start"=array[564 elements], "time_subsample_start"=array[564 elements], "time_FEA_start"=array[564 elements], "time_FEA_end"=array[564 elements], "time_cycle_end"=array[564 elements], "time_accelerometer_aquire_start"=array[564 elements], "time_frequency_calculations_start"=array[564 elements], "time_frequency_calculations_end"=array[564 elements], "measured_pin_location_tt"=array[564 elements], "time_ACC_data_collection_start"=80808.5492656, "time_acceleration_data"=array[564 elements], "estimated_pin_location"=array[564 elements], "scaling_factor_Hz_per_pin_to_frequency_resolution"=nan, "Std_Dev_equale_particles_divided_3"=FALSE, "Auto_FFT_length"=FALSE, "windowed_acc_data"=array1x564[564 elements], "FFT"=array1x564[564 elements]}, "FEA Parameters"={"LEMP"={"Eigenvalues"=array[238 elements], "Square Transpose Eigenvectors"=array238x238[56644 elements], "1/deltaStiff"=1e-16}, "nodes of interest"=[19, 20, 21, 22, 23, 24, 25, 26, 27, 28, 29, 30, 31, 32, 33, 34, 35, 36, 37, 38, 39, 40, 41, 42, 43, 44, 45, 46, 47, 48, 49, 50, 51, 52], "all nodes"=[1, 2, 3, 4, 5, 6, 7, 8, 9, 10, 11, 12, 13, 14, 15, 16, 17, 18, 19, 20, 21, 22, 23, 24, 25, 26, 27, 28, 29, 30, 31, 32, 33, 34, 35, 36, 37, 38, 39, 40, 41, 42, 43, 44, 45, 46, 47, 48, 49, 50, 51, 52, 53, 54, 55, 56, 57, 58, 59, 60, 61, 62, 63, 64, 65, 66, 67, 68, 69, 70, 71, 72, 73, 74, 75, 76, 77, 78, 79, 80, 81, 82, 83, 84, 85, 86, 87, 88, 89, 90, 91, 92, 93, 94, 95, 96, 97, 98, 99, 100, 101, 102, 103, 104, 105, 106, 107, 108, 109, 110, 111, 112, 113, 114, 115, 116, 117, 118, 119], "Eigenvalue Method"=enum."0-Local Eigen Modification Procedure", "Mode Count"=3, "initial_pin_node"=0, "Sub Sample"=TRUE}, "Modeling Parameters"={"beam_length"=0.3525, "youngs_modulus"=209500000000.0, "torsion_spring"=0.0, "beam_height"=0.00635, "beam_width"=0.0508, "beam_density"=7900.0, "number_of_FEA_nodes"=120, "FFT_data_length"=4000, "standard_deviation"=2.0, "number_of_particles"=5, "min_FFT_power_value"=0.02, "initial_pin_node"=0, "accelerometer_mass"=0.055, "Max Roller Velocity"=3.32, "Max frequency delta per second"=-320.2269503546099, "Max frequency delta per node"=-1.0, "Min frequency"=49.84843481411623, "Max frequency"=87.165148551616}}  # Experiment
  n1 = Format Date/Time String() -> (date/time string=w15:string)  [unwired: 3 in]
  n2 = Unbundle(w35) -> ("Experimental Results"=w31:T4, "FEA Parameters"=w33:T5, "Modeling Parameters"=w34:T6)  [unwired: 1 out]
  n3 = Bundle(cluster=w31, "time_average_cycle"=0.0 ("relative seconds"), "measured_frequency"=w1, "date_time"=w15, "time_cycle_start"=w1, "measured_pin_location"=w1, "estimated_frequency"=w1, "acceleration_data"=w1, "time_compare_start"=w1, "time_subsample_start"=w1, "time_FEA_start"=w1, "time_FEA_end"=w1, "time_cycle_end"=w1, "time_accelerometer_aquire_start"=w1, "time_frequency_calculations_start"=w1, "time_frequency_calculations_end"=w1, "measured_pin_location_tt"=w1, "time_acceleration_data"=w1, "estimated_pin_location"=w1, "scaling_factor_Hz_per_pin_to_frequency_resolution"="scaling_factor_Hz_per_pin_to_frequency_resolution", "Std_Dev_equale_particles_divided_3"="Std. Dev = Number of Particles / 3", "Auto_FFT_length"="Auto FFT length", "windowed_acc_data"=w3, "FFT"=w3) -> (w30:T4)  [unwired: 4 in]
  n4 = Bundle(cluster=w34, "beam_length"="Length of Beam", "youngs_modulus"="Young's Modulus", "torsion_spring"="Torsion Spring", "beam_height"="Height", "beam_width"="Width", "beam_density"="Density", "number_of_FEA_nodes"="FEA Nodes", "FFT_data_length"="FFT data length (data points)", "standard_deviation"="Std. Dev.", "number_of_particles"="Number Of Particles", "min_FFT_power_value"="Min. FFT Power Value (RMS)", "initial_pin_node"="Initial Pin node", "accelerometer_mass"="accelerometer_mass", "Max Roller Velocity"="Max Roller Velocity") -> (w36:T6)  [unwired: 4 in]
  n5 = Bundle(cluster=w33, "Sub Sample"="Sub Sample") -> (w32:T5)  [unwired: 6 in]
  n6 = Bundle By Name(cluster=w35, "Experimental Results"=w30, "FEA Parameters"=w32, "Modeling Parameters"=w36) -> (w37:T3)
  n7 = call "Sub_Preprocessing_Main.vi"("Experiment in"=w37) -> ("Experiment out"=w38:T3)  [unwired: 10 in]
  n8 = while "For Loop: Master Loop" {
    shift-right: [w56] -> w10
    shift-left: w38 -> [w69]
    shift-right: [w46] -> _
    shift-left: T2 {"State"=[[0.0], [0.0]], "F state prop matrix"=[[1.0000294843345943, 8.693259864029983e-10], [0.0, 1.0000294843345943]], "H measure matrix"=[[1.0, 0.0], [0.0, 1.0]], "P process cov"=[[0.1, 0.0], [0.0, 0.1]], "R measure cov"=[[0.2]], "Q state cov"=[[0.1, 0.0], [0.0, 0.1]], "T Sample"=2.948389993980527e-05, "New Measurement"=0.058339862830293715, "Measurement Variance"=0.2, "State Variance"=0.1, "Threshold"=0.4, "Initialized"=FALSE} ("KF") -> [w48]
    i -> [w63]
    stop <- w39 stop-if-true
    n9 = Not(x="Loop") -> (.not. x?=w41:bool)
    n10 = call "Sub_Online_FFT.vi"("Bound to 1st Frequency"="Bound to 1st Frequency", "Frequency Method"="Frequency Method", "Experiment in"=w69) -> ("looping"=w43:bool, "Experiment out"=w71:T7)  [unwired: 7 in]
    n11 = And(x=w43, y=w41) -> (x .and. y?=w45:bool)
    n12 = Bundle By Name(cluster=w48, "Threshold"="Threshold", "State Variance"="State Variance", "Measurement Variance"="Measurement Variance") -> (w47:T2)
    n13 = Quotient & Remainder(x=w63, y="Plot Update Frequency") -> (x-y*floor(x/y)=w64:i32)  [unwired: 1 out]
    n14 = Or(x=w45, y="MASTER") -> (x .or. y?=w39:bool)
    n15 = Equal To 0?(x=w64) -> (x = 0?=w61:bool)
    n16 = And(x="Real-Time plotting", y=w61) -> (x .and. y?=w51:bool)
    n17 = Or(x="Pull Plot", y=w51) -> (x .or. y?=w50:bool)
    n18 = call "Sub_Online_FEA.vi"("Bound Search"="Bound Search", "Mode Count"="Mode Count", "Eigenvalue Method"="Eigenvalue Method", "Experiment In"=w71) -> ("Experiment Out"=w60:T3)  [unwired: 7 in]
    n19 = Or(x=w39, y=w50) -> (x .or. y?=w40:bool)
    n20 = case "KF enable" shown="True" "Kalman filter" {
      tunnel: w60 -> [w78 w80]
      tunnel: [w78 w79] -> w52
      tunnel: w47 -> [w77 w82]
      tunnel: [w77 w81] -> w46
      frame False {
      }
      frame True {
        n21 = call "Sub_Kalman_main.vi"("Experiment"=w80, "KF"=w82) -> ("Experiment"=w79:T3, "KF"=w81:T2)  [unwired: 8 in]
      }
    }
    n22 = case "Live Plotting Functions" shown="True" w40 {
      tunnel: w52 -> [_ w86]
      frame False {
      }
      frame True {
        n23 = disable-structure shown="Disabled" {
          frame Disabled {
            n24 = case shown="True" "PDF" {
              tunnel: _ -> [_ w100]
              tunnel: _ -> [_ w99]
              tunnel: _ -> [_ w98]
              tunnel: _ -> [_ w97]
              frame False {
                n25 = Wait (ms)(milliseconds to wait=u32 4) -> ()  [unwired: 1 out]
              }
              frame True {
                n26 = Bundle(w98, w97) -> (→"Probability Density Function":cluster{void, void})  [unwired: 1 in]
                n27 = control-ref of="Probability Density Function"() -> (w94:refnum<vi>)
                n28 = call-poly <vilib>:"Continuous Moments.vi"("std"=w100, "mean"=w99) -> ("variance"=w95:dbl, "mean"=w93:dbl)  [unwired: 7 in, 1 out]
                n29 = call "sub_plot_PDF_in_real_time.vi"("mean"=w93, "variance"=w95, "XYGraph in"=w94) -> ()  [unwired: 9 in]
              }
            }
          }
          frame Enabled {
          }
        }
        n30 = call "Sub_plotter.vi"("Experiment"=w86) -> ("Plotables"=w85:T8)  [unwired: 9 in]
        n31 = Unbundle(w85) -> (→"1st Nat. Freq. (Hz) 2":dbl, "FFT"=→"FFT":dbl[], "Dynamic Data"=→"Frequencies":dynamicdata, "acceleration_data"=→"Acceleration Data":dbl[], →"Cycle time (ms)":dbl, "Dynamic Data"=→"Absolute position":dynamicdata)  [unwired: 1 out]
      }
    }
    n32 = case shown="True" TRUE {
      tunnel: [w73 w76] -> w56
      tunnel: w52 -> [w73 w75]
      tunnel: "Truncate data length" -> [_ w74]
      frame False {
      }
      frame True {
        n33 = call "Sub_Truncate_dataset.vi"("Truncate data length"=w74, "Experiment"=w75) -> ("Experiment"=w76:T3)  [unwired: 9 in]
      }
    }
  }
  n34 = call "Sub_post_processing.vi"("Experiment"=w10, "file name"="File name", "Save Acceleration Data"="Save Acceleration Data") -> ("Frequency"=→"Frequency space":waveform(dbl)[], "Position"=→"Position Pinned Boundary condition":waveform(dbl)[], "average cycle time (s)"=→"average cycle time (s)":dbl)  [unwired: 5 in]
